vi "HTML Report Labeled Numeric Table.vi"(0 "Show Grid":bool, 2 "column width (100)":dbl=100.0, 4 "format (%f)":string="%f", 5 "width":string, 6 "align (default)":T1, 7 "transpose array (F)":bool, 8 "row headers":string[](array[string]), 9 "column headers":string[](array[string]), 10 "table contents":dbl[][](array[numeric]) format="%.2f", 11 "HTML in":string) -> (3 "HTML out":string)   [LabVIEW 2020, in "NI_ReportGenerationCore.lvlib"]
doc: "Constructs HTML code to describe a table containing table contents, row headers and column headers."
uses:
  NI_ReportGenerationCore.lvlib
  HTML Report Text Alignment.ctl
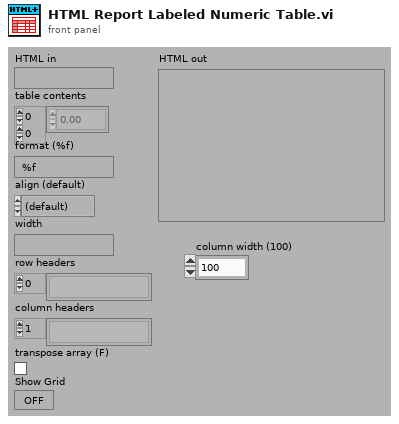
[diagram p1: front panel]
types:
  T1 = typedef "NI_ReportGenerationCore.lvlib/HTML Report Text Alignment.ctl" = enum16{"(default)", "LEFT", "CENTER", "RIGHT"}
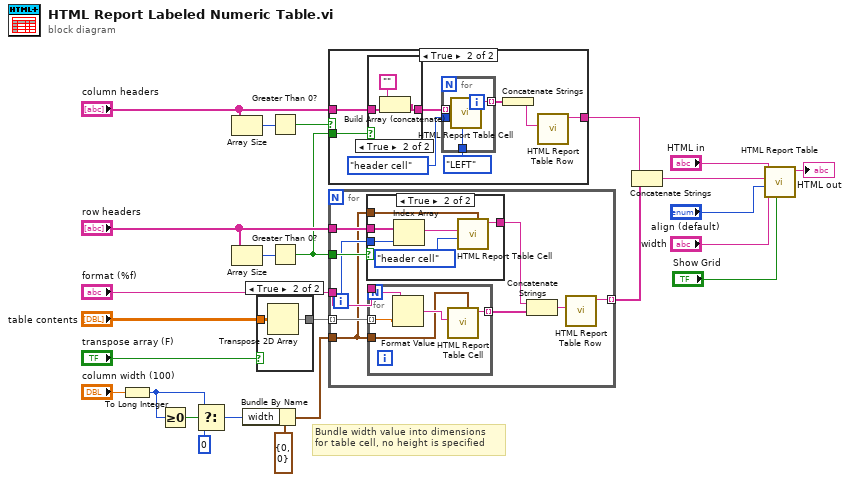
[diagram p0: block diagram]
diagram:
  # "Bundle width value into dimensions\nfor table cell, no height is specified"
  n1 = To Long Integer(number="column width (100)") -> (32bit integer=w2:i32)
  n2 = Greater Or Equal To 0?(x=w2) -> (x >= 0?=w4:bool)
  n3 = Select(t=w2, s=w4, f=0 ("32bit integer")) -> (s? t:f=w1:i32)
  n4 = Array Size(array="column headers") -> (size(s)=w18:i32)
  n5 = Array Size(array="row headers") -> (size(s)=w14:i32)
  n6 = Bundle By Name(cluster=cluster{"height":i32, "width":i32} {"height"=0, "width"=0} ("pixel size (default)"), "width"=w1) -> (w5:cluster{"height":i32, "width":i32})
  n7 = case shown="True" "transpose array (F)" {
    tunnel: "table contents" -> [w26 w28]
    tunnel: [w26 w27] -> w19
    frame False {
    }
    frame True {
      n8 = Transpose 2D Array(2D array=w28) -> (transposed array=w27:dbl[][])
    }
  }
  n9 = Greater Than 0?(x=w18) -> (x > 0?=w16:bool)
  n10 = Greater Than 0?(x=w14) -> (x > 0?=w12:bool)
  n11 = case shown="True" w16 {
    tunnel: "column headers" -> [_ w30]
    tunnel: [_ w33] -> w15
    tunnel: w12 -> [_ w32]
    frame False {
    }
    frame True {
      n12 = case shown="True" w32 {
        tunnel: w30 -> [w37 w40]
        tunnel: [w37 w39] -> w31
        frame False {
        }
        frame True {
          n13 = Build Array (concatenate)("" ("Empty String Constant"), w40) -> (w39:string[])
        }
      }
      n14 = for {
        tunnel: [w44] -> w36 mode=indexing
        tunnel: enum16{"data cell", "header cell"}."header cell" ("cell type (data cell)") -> [w43]
        tunnel: w31 -> [w42] mode=indexing
        tunnel: HTML_Report_Text_Alignment."LEFT" ("align (default)") -> [w41]
        n15 = call "HTML Report Table Cell.vi"("align (default)"=w41, "cell type (data cell)"=w43, "cell contents"=w42) -> ("table cells out"=w44:string)  [unwired: 1 in, 7 out]
      }
      n16 = Concatenate Strings(w36) -> (w34:string)
      n17 = call "HTML Report Table Row.vi"("table cells"=w34) -> ("table rows out"=w33:string)  [unwired: 1 in, 5 out]
    }
  }
  n18 = for {
    tunnel: w19 -> [w54] mode=indexing
    tunnel: [w51] -> w25 mode=indexing
    tunnel: w12 -> [w50]
    tunnel: "row headers" -> [w49]
    tunnel: "format (%f)" -> [w46]
    tunnel: w5 -> [w45]
    i -> [w48]
    n19 = case shown="True" w50 {
      tunnel: w49 -> [_ w60]
      tunnel: w48 -> [_ w59]
      tunnel: [_ w56] -> w47
      tunnel: w45 -> [_ w55]
      frame False {
      }
      frame True {
        n20 = Index Array(array=w60, index=w59) -> (element=w58:string)
        n21 = call "HTML Report Table Cell.vi"("pixel size (default)"=w55, "cell type (data cell)"=enum16{"data cell", "header cell"}."header cell", "cell contents"=w58) -> ("table cells out"=w56:string)  [unwired: 1 in, 7 out]
      }
    }
    n22 = for {
      tunnel: w54 -> [w64] mode=indexing
      tunnel: [w65] -> w53 mode=indexing
      tunnel: w46 -> [w62]
      tunnel: w45 -> [w61]
      n23 = Format Value(format string=w62, value (0)=w64) -> (output string=w63:string)  [unwired: 1 out]
      n24 = call "HTML Report Table Cell.vi"("pixel size (default)"=w61, "cell contents"=w63) -> ("table cells out"=w65:string)  [unwired: 1 in, 8 out]
    }
    n25 = Concatenate Strings(w47, w53) -> (w52:string)
    n26 = call "HTML Report Table Row.vi"("table cells"=w52) -> ("table rows out"=w51:string)  [unwired: 1 in, 5 out]
  }
  n27 = Concatenate Strings(w15, w25) -> (w24:string)
  n28 = call "HTML Report Table.vi"("Show Grid"="Show Grid", "width"="width", "align (default)"="align (default)", "table rows"=w24, "HTML in"="HTML in") -> ("HTML out"=→"HTML out":string)  [unwired: 3 out]
